vi "Host_Main.vi"() -> ()   [LabVIEW 2016]
uses:
  Application Control/FSM States.ctl
  Application Control/FSM Queue/FSM Data.ctl
  HostRTCommunication/Commands.ctl
  Raw Data/LoggingCommands.ctl
  Application Control/Application Globals.vi
panel:
  in  "Record Button":bool
  in  "Pause Button":bool
  in  "Configuration Cluster":T1={"Center Frequency"=50000000, "Sample Rate (Bandwidth)"=225001, "Tuner AGC Mode"=FALSE, "AGC Mode"=FALSE, "Manual Gain"=0, "Number of Averages"=4, "Frequency Correction"=0} {"Manual Gain" items=["0.000000", "0.900000", "1.400000", "2.700000", "3.700000", "7.700000", "8.700000", "12.500000", "14.400000", "15.700000", "16.600000", "19.700000", "20.700000", "22.900000", "25.400000", "28.000000", "29.700000", "32.800000", "33.800000", "36.400000", "37.200000", "38.600000", "40.200000", "42.100000", "43.400000", "43.900000", "44.500000", "48.000000", "49.600000"]; "Number of Averages" min=1 max=65536 step=1; "Sample Rate (Bandwidth)" min=225001 max=3200000 step=1; "Center Frequency" min=50000000 max=1800000000 step=1}
  in  "Connect":bool
  out "Spectrum Graph":dbl[](graph)
  out "Intensity Graph":dbl[][](graph)
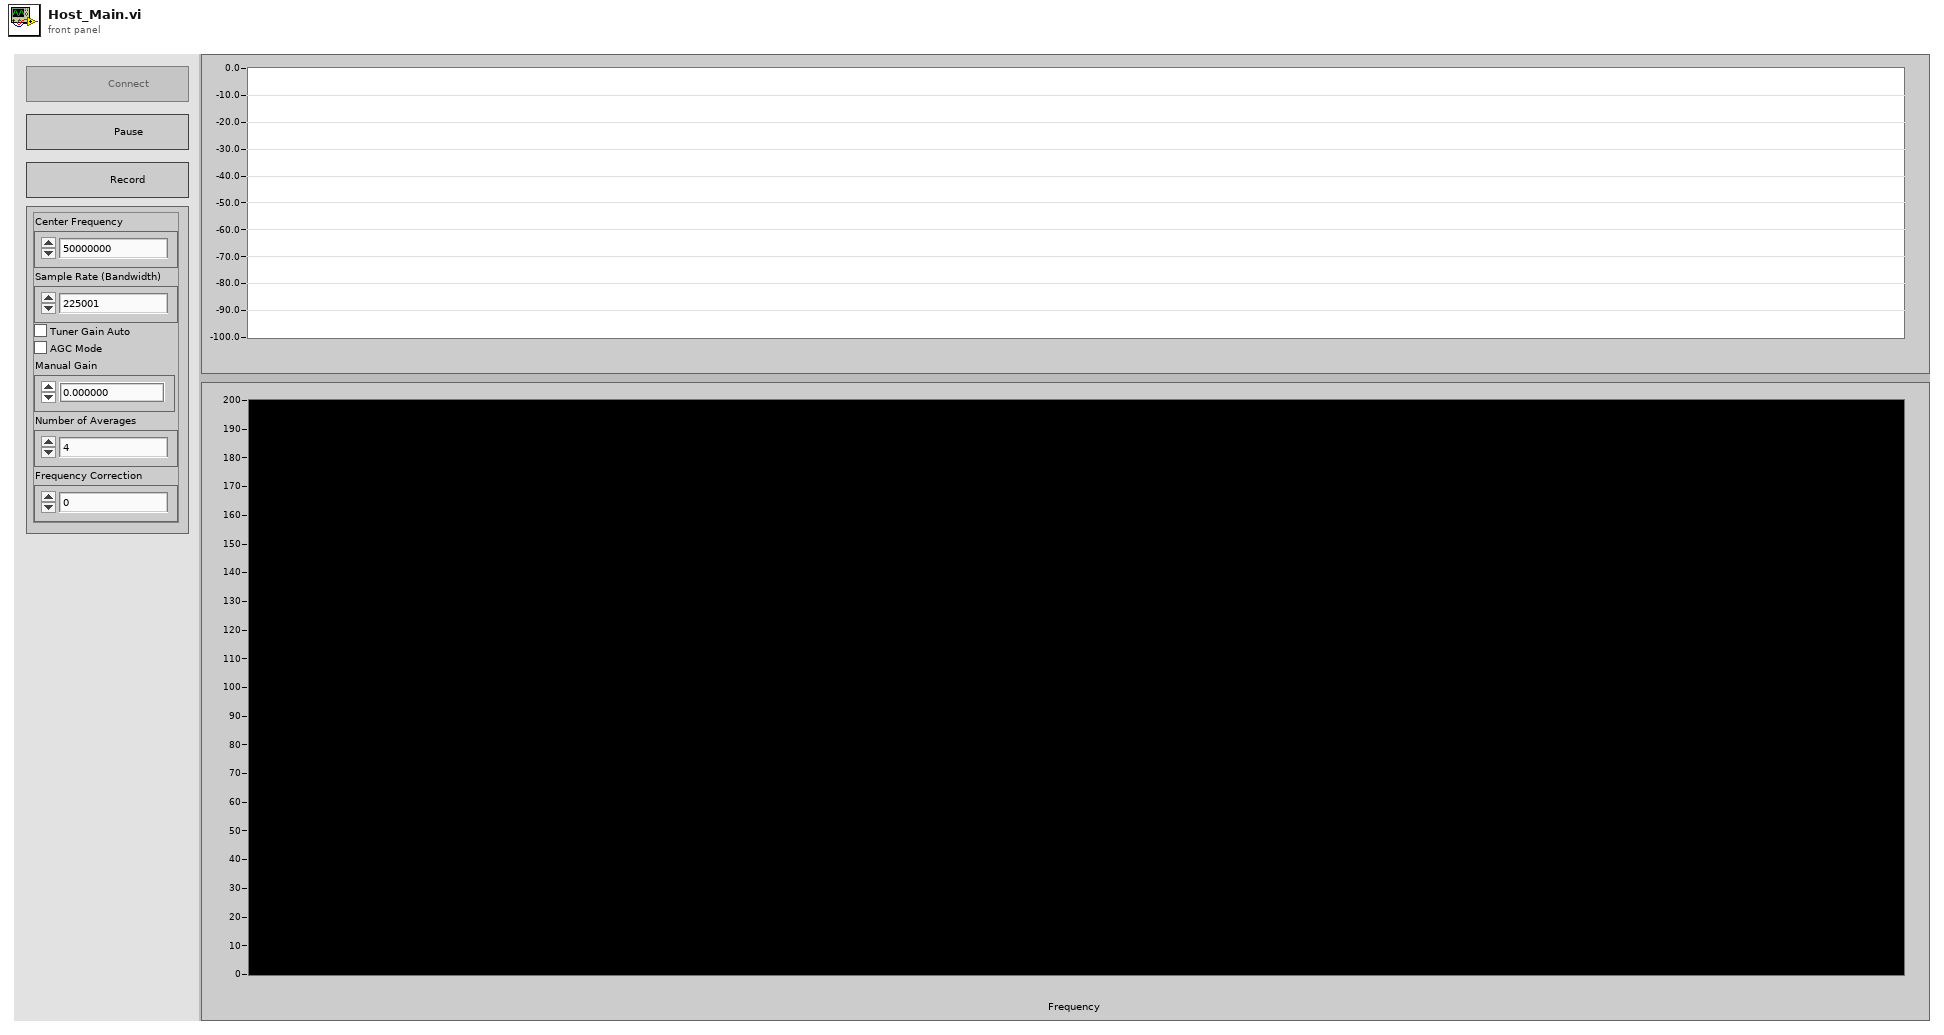
[diagram p1: front panel]
types:
  T1 = cluster{"Center Frequency":u32, "Sample Rate (Bandwidth)":u32, "Tuner AGC Mode":bool, "AGC Mode":bool, "Manual Gain":u16, "Number of Averages":u32, "Frequency Correction":i32}
  T2 = typedef "FSM Data.ctl" = cluster{"FSM State":T3, "Spectrum Reader":refnum<k21>, "Recording":bool, "IP Address":string, "Raw Data Reader":refnum<k21>}
  T3 = typedef "FSM States.ctl" = enum16{"App_Idle", "App_Connect", "App_Close", "APP_Init", "App_Logging", "App_SetRecordStateOn", "App_SetRecordStateOff"}
  T4 = enum8{"Enabled", "Disabled", "Disabled and Grayed Out"}
  T5 = typedef "LoggingCommands.ctl" = enum16{"Write", "Close File", "Open File", "Set Channel Metadata"}
  T6 = typedef "Commands.ctl" = enum16{"Set Center Frequency", "Set AGC State", "Set Number Of Averages", "Set Tuner Gain Mode", "Set Frequency Correction", "Set Sample Rate", "Set Manual Gain Value"}
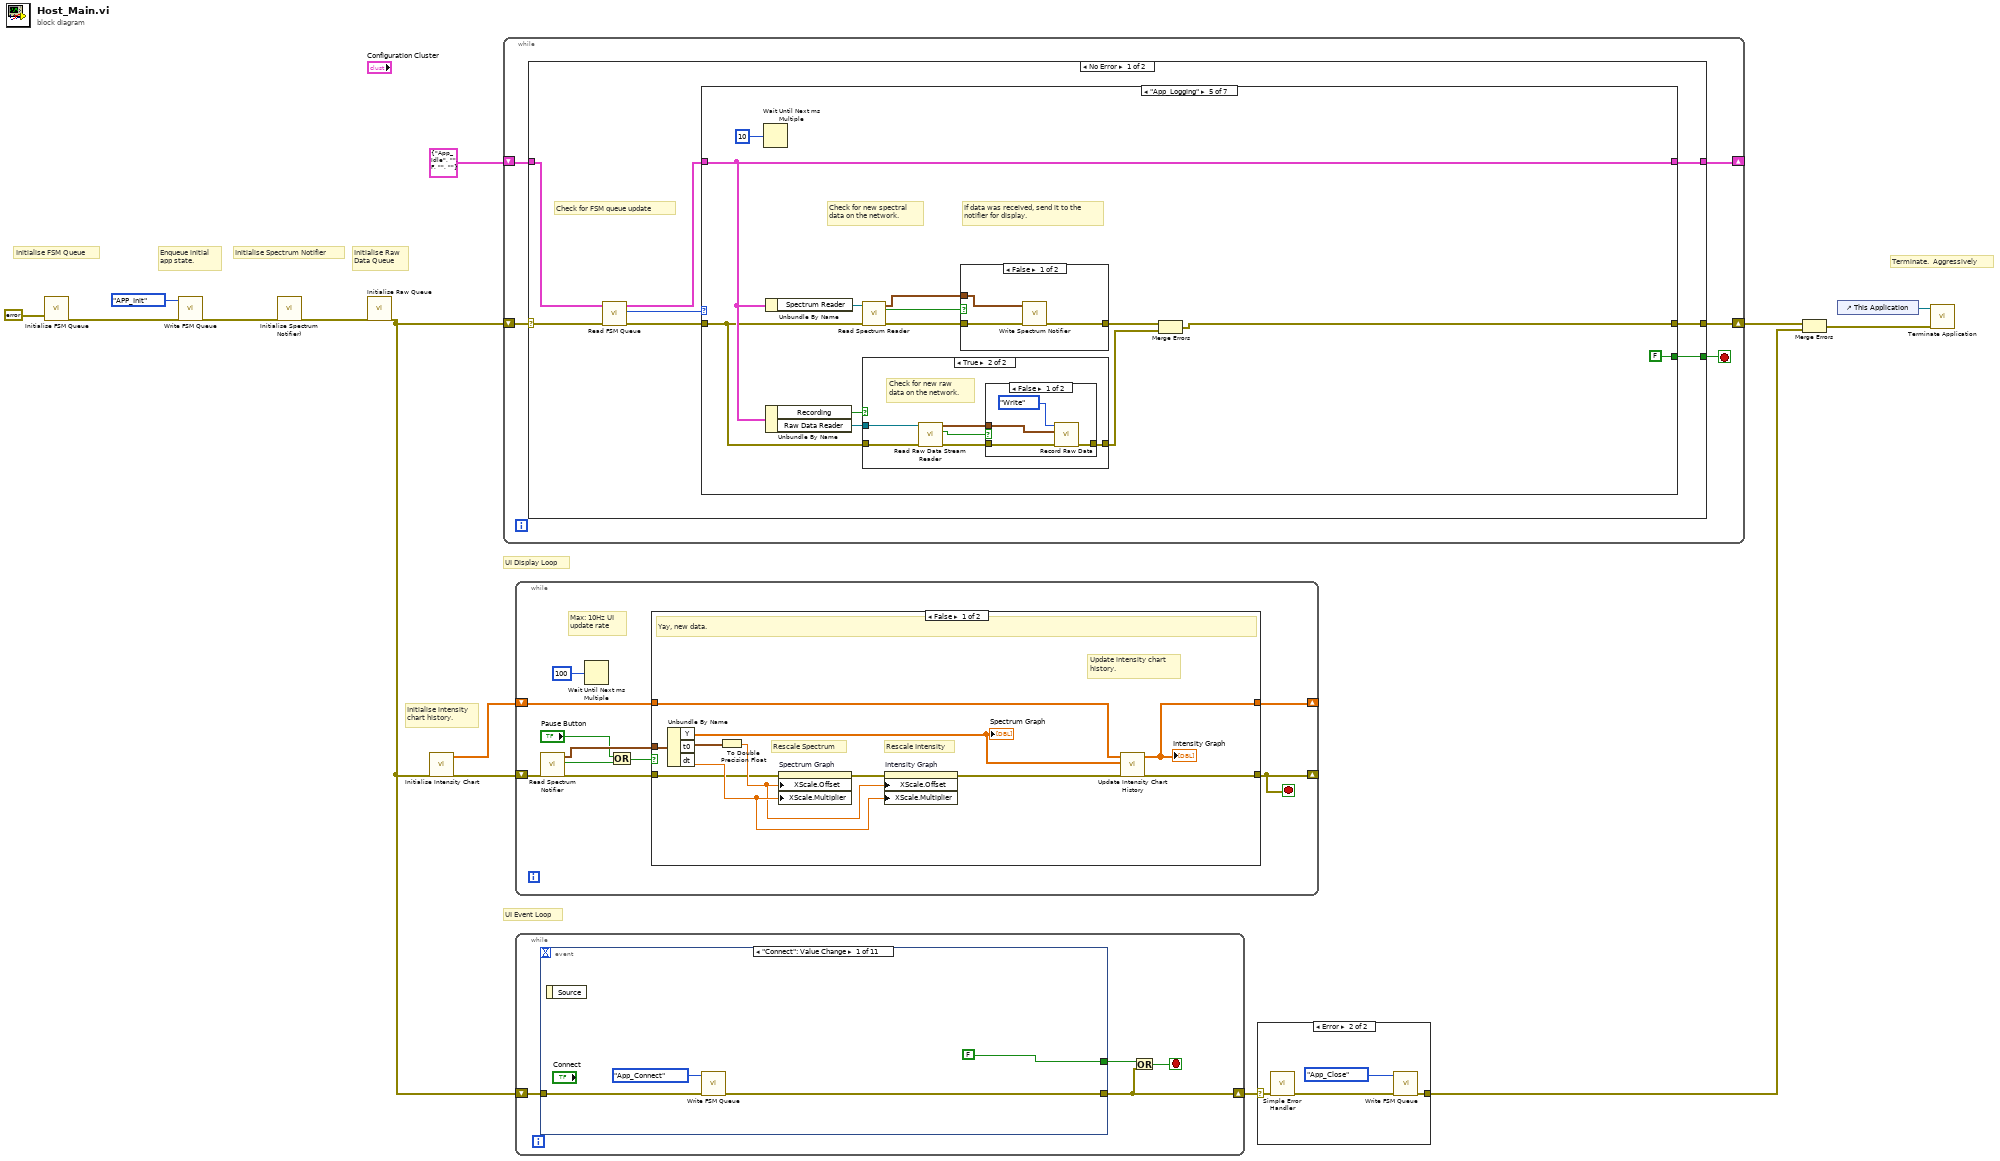
[diagram p0: block diagram]
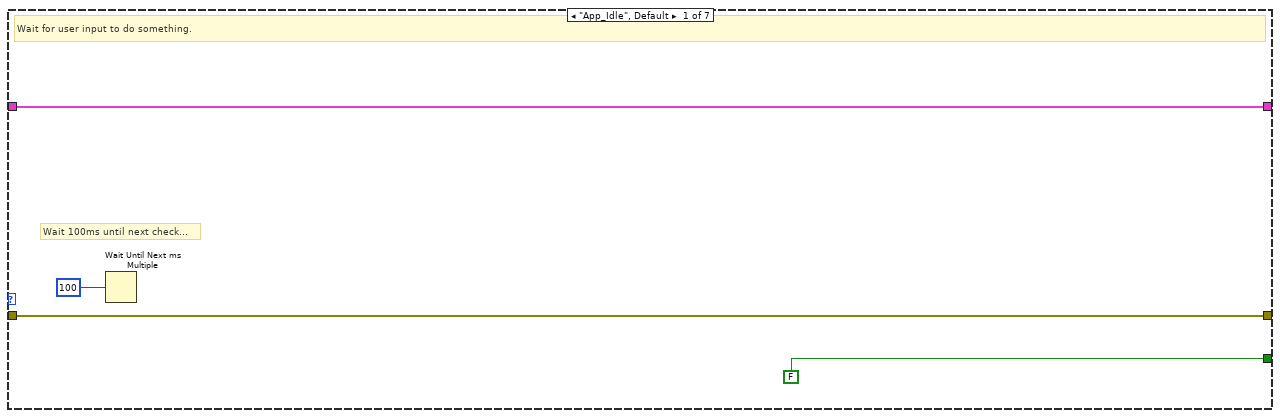
[diagram p2: hidden frame]
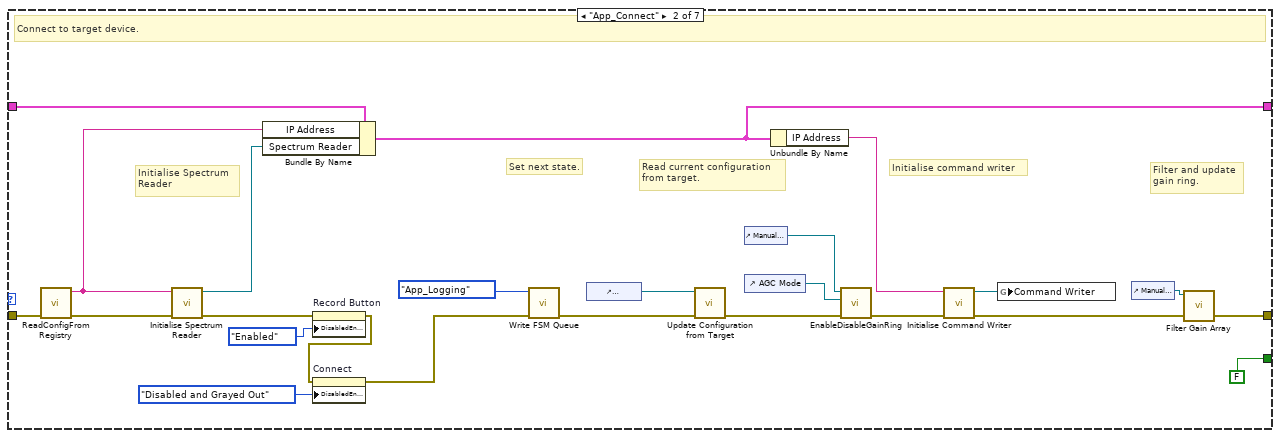
[diagram p3: hidden frame]
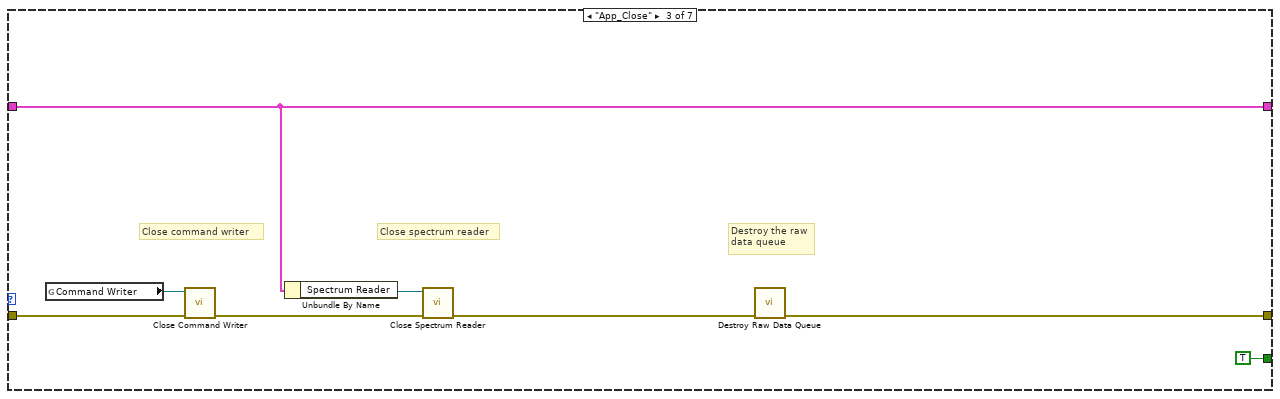
[diagram p4: hidden frame]
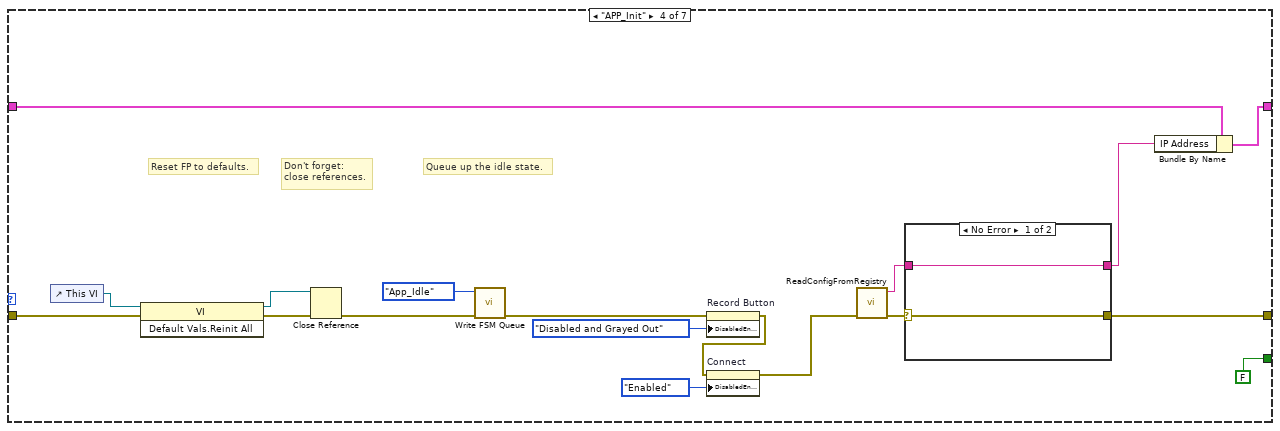
[diagram p5: hidden frame]
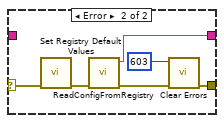
[diagram p6: hidden frame]
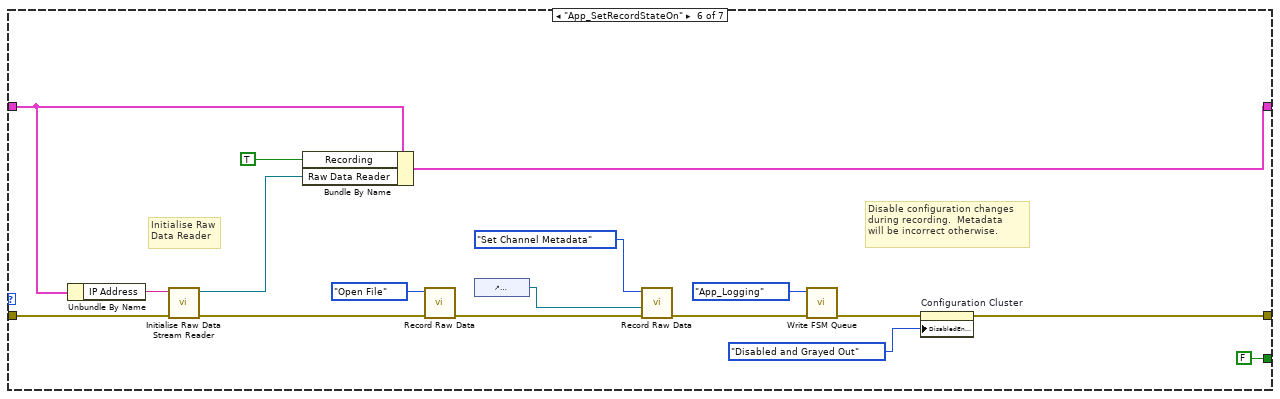
[diagram p10: hidden frame]
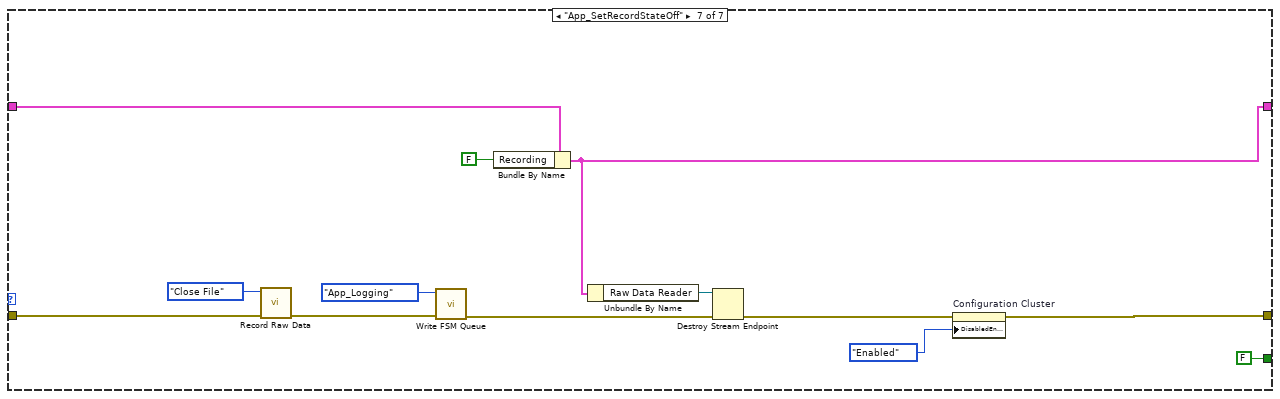
[diagram p11: hidden frame]
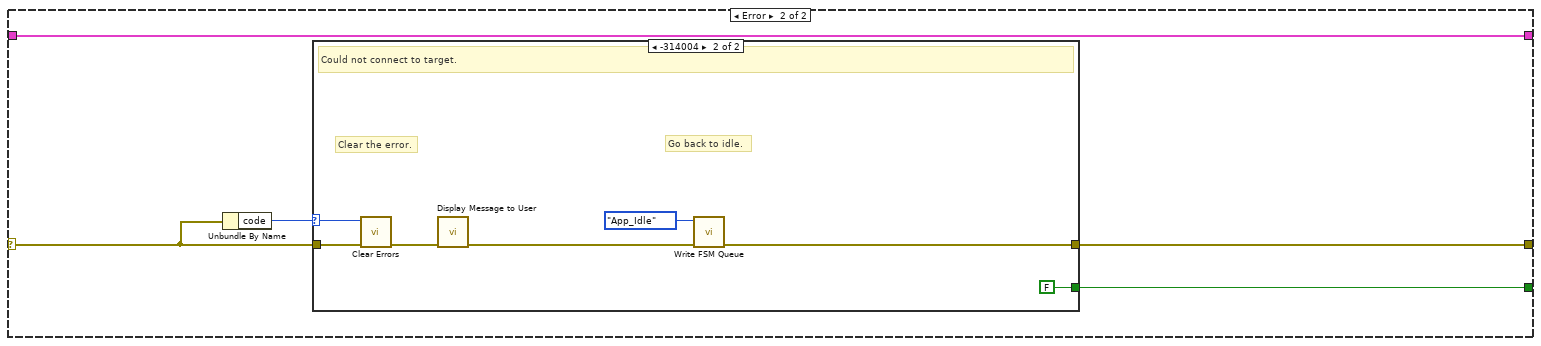
[diagram p12: hidden frame]
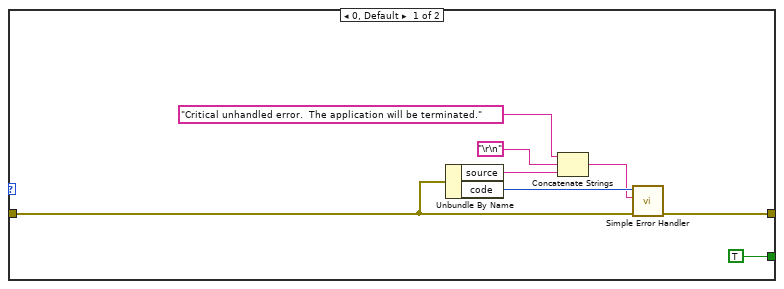
[diagram p13: hidden frame]
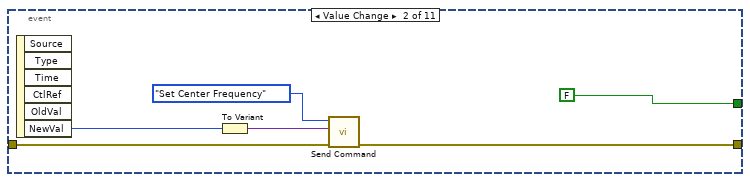
[diagram p16: hidden frame]
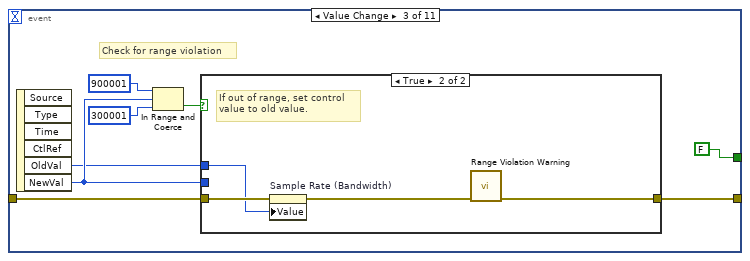
[diagram p17: hidden frame]
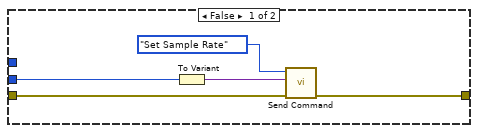
[diagram p18: hidden frame]
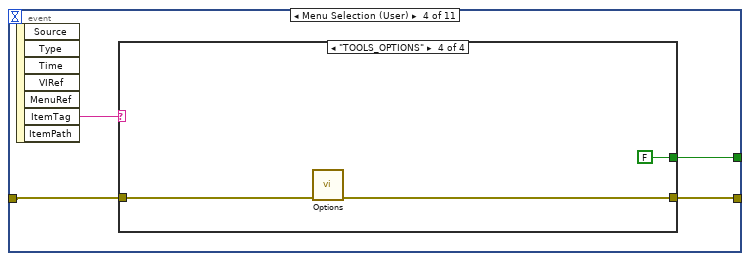
[diagram p19: hidden frame]
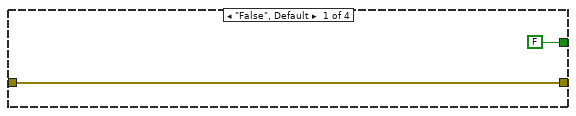
[diagram p20: hidden frame]
diagram:
  # "Initialise Raw\nData Queue"
  # "Initialise intensity\nchart history."
  # "UI Display Loop"
  # "Initialise Spectrum Notifier"
  # "Terminate.  Aggressively"
  # "Enqueue initial\napp state."
  # "Initialise FSM Queue"
  # "UI Event Loop"
  n1 = call "Initialise FSM Queue.vi"("error in (no error)"=errorcluster {"status"=FALSE, "code"=0, "source"=""}) -> ("error out"=w13:errorcluster)  [unwired: 10 in]
  n2 = call "Write FSM Queue.vi"("error in (no error)"=w13, "App_State"=FSM_States."APP_Init") -> ("error out"=w10:errorcluster)  [unwired: 9 in]
  n3 = call "Initialise Spectrum Notifier).vi"("error in (no error)"=w10) -> ("error out"=w3:errorcluster)  [unwired: 10 in]
  n4 = call "Initialise Raw Queue.vi"("error in (no error)"=w3) -> ("error out"=w1:errorcluster)  [unwired: 10 in]
  n5 = call "Initialise Intensity Chart.vi"("error in (no error)"=w1) -> ("error out"=w8:errorcluster, "Array"=w9:dbl[][])  [unwired: 9 in]
  n6 = while {
    shift-right: [w18] -> _
    shift-left: T2 {"FSM State"=enum."App_Idle", "Spectrum Reader"="", "Recording"=FALSE, "IP Address"="", "Raw Data Reader"=""} ("FSM Data") -> [w19]
    shift-right: [w17] -> w6
    shift-left: w1 -> [w16]
    stop <- w15 stop-if-true
    n7 = case shown="No Error" w16 {
      selector: w16 -> [w23 w151]
      tunnel: w19 -> [w27 w153]
      tunnel: [w21 w153] -> w18
      tunnel: [w24 w149] -> w17
      tunnel: [w20 w150] -> w15
      frame No Error {
        # "Check for FSM queue update"
        n8 = call "Read FSM Queue.vi"("error in (no error)"=w23, "FSM Data in"=w27) -> ("error out"=w25:errorcluster, "FSM State"=w26:T3, "FSM Data out"=w22:T2)  [unwired: 7 in]
        n9 = case shown="\"App_Logging\"" w26 {
          tunnel: w25 -> [w31 w36 w62 w79 w95 w131 w145]
          tunnel: [w31 w48 w57 w64 w92 w120 w136] -> w24
          tunnel: w22 -> [w30 w42 w58 w67 w97 w129 w147]
          tunnel: [w30 w33 w58 w65 w97 w134 w142] -> w21
          tunnel: [FALSE FALSE TRUE FALSE FALSE FALSE FALSE] -> w20
          frame "App_Idle", Default {
            # "Wait 100ms until next check..."
            # "Wait for user input to do something."
            n10 = Wait Until Next ms Multiple(millisecond multiple=u32 100) -> ()  [unwired: 1 out]
          }
          frame "App_Connect" {
            # "Initialise Spectrum \nReader"
            # "Filter and update\ngain ring."
            # "Initialise command writer"
            # "Read current configuration\nfrom target."
            # "Set next state."
            # "Connect to target device."
            n11 = call "ReadConfigFromRegistry.vi"("error in (no error)"=w36) -> ("error out"=w35:errorcluster, "String/Binary data"=w34:string)  [unwired: 9 in]
            n12 = call "Initialise Spectrum Reader.vi"("error in (no error)"=w35, "IP Address"=w34) -> ("error out"=w41:errorcluster, "Spectrum Reader"=w55:refnum<k21>)  [unwired: 8 in]
            n13 = Bundle By Name(cluster=w42, "IP Address"=w34, "Spectrum Reader"=w55) -> (w33:T2)
            n14 = property on="Record Button" class="Bool (strict)"(error in=w41, "DisabledEnum"=T4."Enabled" ("Disabled")) -> (error out=w38:errorcluster)  [unwired: 1 in, 1 out]
            n15 = property on="Connect" class="Bool"(error in=w38, "DisabledEnum"=T4."Disabled and Grayed Out" ("Disabled")) -> (error out=w37:errorcluster)  [unwired: 1 in, 1 out]
            n16 = call "Write FSM Queue.vi"("error in (no error)"=w37, "App_State"=FSM_States."App_Logging") -> ("error out"=w52:errorcluster)  [unwired: 9 in]
            n17 = control-ref of="Configuration Cluster"() -> (w50:refnum<vi>)
            n18 = call "Update Configuration from Target.vi"("error in (no error)"=w52, "Configuration Cluster"=w50) -> ("error out"=w46:errorcluster)  [unwired: 9 in]
            n19 = control-ref of="Manual Gain"() -> (w44:refnum<vi>)
            n20 = control-ref of="AGC Mode"() -> (w43:refnum<vi>)
            n21 = Unbundle By Name(w33) -> ("IP Address"=w32:string)
            n22 = call "EnableDisableGainRing.vi"("error in (no error)"=w46, "Bool Refnum"=w43, "Ring in"=w44) -> ("error out"=w45:errorcluster)  [unwired: 8 in]
            n23 = call "Initialise Command Writer.vi"("error in (no error)"=w45, "IP Address"=w32) -> ("error out"=w49:errorcluster, "Refnum out"=w51:refnum<k21>)  [unwired: 8 in]
            n24 = global write "Application Globals.vi" "Command Writer"(w51) -> ()
            n25 = control-ref of="Manual Gain"() -> (w47:refnum<vi>)
            n26 = call "Filter Gain Array.vi"("error in (no error)"=w49, "Gain Ring Reference"=w47) -> ("error out"=w48:errorcluster)  [unwired: 9 in]
          }
          frame "App_Close" {
            # "Destroy the raw\ndata queue"
            # "Close spectrum reader"
            # "Close command writer"
            n27 = global read "Application Globals.vi" "Command Writer"() -> (w61:refnum<k21>)
            n28 = call "Close Command Writer.vi"("error in (no error)"=w62, "Refnum in"=w61) -> ("error out"=w60:errorcluster)  [unwired: 9 in]
            n29 = Unbundle By Name(w58) -> ("Spectrum Reader"=w59:refnum<k21>)
            n30 = call "Close Spectrum Reader.vi"("error in (no error)"=w60, "endpoint in"=w59) -> ("error out"=w56:errorcluster)  [unwired: 9 in]
            n31 = call "Destroy Raw Data Queue.vi"("error in (no error)"=w56) -> ("error out"=w57:errorcluster)  [unwired: 10 in]
          }
          frame "APP_Init" {
            # "Queue up the idle state."
            # "Don't forget:\nclose references."
            # "Reset FP to defaults."
            n32 = control-ref of="This VI"() -> (w80:refnum<vi>)
            n33 = invoke class="VI" method="Default Vals.Reinit All"(reference=w80, error in=w79) -> (reference out=w76:refnum<vi>, error out=w78:errorcluster)  [unwired: 1 in, 1 out]
            n34 = Close Reference(reference=w76, error in (no error)=w78) -> (error out=w77:errorcluster)
            n35 = call "Write FSM Queue.vi"("error in (no error)"=w77, "App_State"=FSM_States."App_Idle") -> ("error out"=w74:errorcluster)  [unwired: 9 in]
            n36 = property on="Record Button" class="Bool (strict)"(error in=w74, "DisabledEnum"=T4."Disabled and Grayed Out" ("Disabled")) -> (error out=w72:errorcluster)  [unwired: 1 in, 1 out]
            n37 = property on="Connect" class="Bool"(error in=w72, "DisabledEnum"=T4."Enabled" ("Disabled")) -> (error out=w69:errorcluster)  [unwired: 1 in, 1 out]
            n38 = call "ReadConfigFromRegistry.vi"("error in (no error)"=w69) -> ("error out"=w70:errorcluster, "String/Binary data"=w68:string)  [unwired: 9 in]
            n39 = case shown="No Error" w70 {
              selector: w70 -> [w82 w89]
              tunnel: [w83 w87] -> w66
              tunnel: w68 -> [w83 _]
              tunnel: [w82 w84] -> w64
              frame No Error {
              }
              frame Error {
                n40 = call "Set Registry Default Values.vi"("error in (no error)"=w89) -> ("error out"=w88:errorcluster)  [unwired: 10 in]
                n41 = call "ReadConfigFromRegistry.vi"("error in (no error)"=w88) -> ("error out"=w86:errorcluster, "String/Binary data"=w87:string)  [unwired: 9 in]
                n42 = call <vilib>:"Clear Errors.vi"("error in (no error)"=w86, "specific error code to clear (0: all)"=603) -> ("error out"=w84:errorcluster)  [unwired: 4 in, 1 out]
              }
            }
            n43 = Bundle By Name(cluster=w67, "IP Address"=w66) -> (w65:T2)
          }
          frame "App_Logging" {
            # "If data was received, send it to the\nnotifier for display."
            # "Check for new spectral\ndata on the network."
            n44 = Wait Until Next ms Multiple(millisecond multiple=u32 10) -> ()  [unwired: 1 out]
            n45 = Unbundle By Name(w97) -> ("Spectrum Reader"=w102:refnum<k21>)
            n46 = Unbundle By Name(w97) -> ("Recording"=w90:bool, "Raw Data Reader"=w96:refnum<k21>)
            n47 = call "Read Spectrum Reader.vi"("error in (no error)"=w95, "Refnum in"=w102) -> ("error out"=w99:errorcluster, "Boolean"=w100:bool, "output waveform"=w98:waveform(dbl))  [unwired: 7 in]
            n48 = case shown="True" w90 {
              tunnel: w96 -> [_ w109]
              tunnel: w95 -> [w103 w108]
              tunnel: [w103 w106] -> w93
              frame False {
              }
              frame True {
                # "Check for new raw\ndata on the network."
                n49 = call "Read Raw Data Stream Reader.vi"("error in (no error)"=w108, "Raw Data Reader"=w109) -> ("error out"=w107:errorcluster, "timed out?"=w104:bool, "Output Waveform"=w105:waveform(u8))  [unwired: 7 in]
                n50 = case shown="False" w104 {
                  tunnel: w107 -> [w113 w114]
                  tunnel: [w112 w114] -> w106
                  tunnel: w105 -> [w111 _]
                  frame False {
                    n51 = call "Record Raw Data.vi"("error in (no error)"=w113, "Raw Data"=w111, "Command"=LoggingCommands."Write") -> ("error out"=w112:errorcluster)  [unwired: 8 in]
                  }
                  frame True {
                  }
                }
              }
            }
            n52 = case shown="False" w100 {
              tunnel: [w117 w118] -> w94
              tunnel: w99 -> [w115 w118]
              tunnel: w98 -> [w116 _]
              frame False {
                n53 = call "Write Spectrum Notifier.vi"("error in (no error)"=w115, "Waveform"=w116) -> ("error out"=w117:errorcluster)  [unwired: 9 in]
              }
              frame True {
              }
            }
            n54 = Merge Errors(w94, w93) -> (w92:errorcluster)
          }
          frame "App_SetRecordStateOn" {
            # "Disable configuration changes\nduring recording.  Metadata\nwill be incorrect otherwise."
            # "Initialise Raw\nData Reader"
            n55 = Unbundle By Name(w129) -> ("IP Address"=w128:string)
            n56 = call "Initialise Raw Data Stream Reader.vi"("error in (no error)"=w131, "IP Address"=w128) -> ("error out"=w130:errorcluster, "reader endpoint"=w127:refnum<k21>)  [unwired: 8 in]
            n57 = Bundle By Name(cluster=w129, "Recording"=TRUE, "Raw Data Reader"=w127) -> (w134:T2)
            n58 = call "Record Raw Data.vi"("error in (no error)"=w130, "Command"=LoggingCommands."Open File") -> ("error out"=w125:errorcluster)  [unwired: 9 in]
            n59 = control-ref of="Configuration Cluster"() -> (w122:refnum<vi>)
            n60 = call "Record Raw Data.vi"("error in (no error)"=w125, "Configuration Cluster"=w122, "Command"=LoggingCommands."Set Channel Metadata") -> ("error out"=w124:errorcluster)  [unwired: 8 in]
            n61 = call "Write FSM Queue.vi"("error in (no error)"=w124, "App_State"=FSM_States."App_Logging") -> ("error out"=w121:errorcluster)  [unwired: 9 in]
            n62 = property on="Configuration Cluster" class="Clust (strict)"(error in=w121, "DisabledEnum"=T4."Disabled and Grayed Out" ("Disabled")) -> (error out=w120:errorcluster)  [unwired: 1 in, 1 out]
          }
          frame "App_SetRecordStateOff" {
            n63 = call "Record Raw Data.vi"("error in (no error)"=w145, "Command"=LoggingCommands."Close File") -> ("error out"=w144:errorcluster)  [unwired: 9 in]
            n64 = call "Write FSM Queue.vi"("error in (no error)"=w144, "App_State"=FSM_States."App_Logging") -> ("error out"=w141:errorcluster)  [unwired: 9 in]
            n65 = Bundle By Name(cluster=w147, "Recording"=FALSE) -> (w142:T2)
            n66 = Unbundle By Name(w142) -> ("Raw Data Reader"=w140:refnum<k21>)
            n67 = Destroy Stream Endpoint(8:w141, 11:w140) -> (0:w137:errorcluster)
            n68 = property on="Configuration Cluster" class="Clust (strict)"(error in=w137, "DisabledEnum"=T4."Enabled" ("Disabled")) -> (error out=w136:errorcluster)  [unwired: 1 in, 1 out]
          }
        }
      }
      frame Error {
        n69 = Unbundle By Name(w151) -> ("code"=w152:i32)
        n70 = case shown="-314004" w152 {
          selector: w152 -> [_ w166]
          tunnel: w151 -> [w160 w167]
          tunnel: [TRUE FALSE] -> w150
          tunnel: [w154 w162] -> w149
          frame 0, Default {
            n71 = Unbundle By Name(w160) -> ("source"=w158:string, "code"=w159:i32)
            n72 = Concatenate Strings("Critical unhandled error.  The application will be terminated.", "\r\n", w158) -> (w155:string)
            n73 = call <vilib>:"Simple Error Handler.vi"("error code (no error:0)"=w159, "error source (\" \")"=w155, "error in (no error)"=w160) -> ("error out"=w154:errorcluster)  [unwired: 2 in, 4 out]
          }
          frame -314004 {
            # "Go back to idle."
            # "Clear the error."
            # "Could not connect to target."
            n74 = call <vilib>:"Clear Errors.vi"("error in (no error)"=w167, "specific error code to clear (0: all)"=w166) -> ("error out"=w165:errorcluster)  [unwired: 4 in, 1 out]
            n75 = call "Display Message to User"("error in (no error)"=w165) -> ("error out"=w163:errorcluster)  [unwired: 9 in, 1 out]
            n76 = call "Write FSM Queue.vi"("error in (no error)"=w163, "App_State"=FSM_States."App_Idle") -> ("error out"=w162:errorcluster)  [unwired: 9 in]
          }
        }
      }
    }
  }
  n77 = while {
    shift-right: [w172] -> _
    shift-left: w8 -> [w178]
    shift-right: [w174] -> _
    shift-left: w9 -> [w175]
    stop <- w172 stop-if-true
    # "Max: 10Hz UI \nupdate rate"
    n78 = call "Read Spectrum Notifier.vi"("error in (no error)"=w178) -> ("error out"=w177:errorcluster, "timed out?"=w171:bool, "WaveForm Out"=w176:waveform(dbl))  [unwired: 8 in]
    n79 = Wait Until Next ms Multiple(millisecond multiple=u32 100) -> ()  [unwired: 1 out]
    n80 = Or(x="Pause Button", y=w171) -> (x .or. y?=w170:bool)
    n81 = case shown="False" w170 {
      tunnel: [w186 w191] -> w172
      tunnel: w177 -> [w180 w191]
      tunnel: w176 -> [w189 _]
      tunnel: w175 -> [w188 w190]
      tunnel: [w187 w190] -> w174
      frame False {
        # "Rescale Intensity"
        # "Rescale Spectrum"
        # "Update intensity chart\nhistory."
        # "Yay, new data."
        n82 = Unbundle By Name(w189) -> ("Y"=w179:dbl[], "t0"=w184:timestamp, "dt"=w183:dbl)
        "Spectrum Graph" <- w179
        n83 = To Double Precision Float(number=w184) -> (double precision float=w182:dbl)
        n84 = property on="Spectrum Graph" class="WFGraph (strict)"(error in=w180, "XScale.Offset"=w182, "XScale.Multiplier"=w183) -> (error out=w181:errorcluster)  [unwired: 1 in, 1 out]
        n85 = property on="Intensity Graph" class="IntGraph (strict)"(error in=w181, "XScale.Offset"=w182, "XScale.Multiplier"=w183) -> (error out=w185:errorcluster)  [unwired: 1 in, 1 out]
        n86 = call "Update Intensity Chart History.vi"("error in (no error)"=w185, "Y"=w179, "Array in"=w188) -> ("error out"=w186:errorcluster, "Array out"=w187:dbl[][])  [unwired: 7 in]
        "Intensity Graph" <- w187
      }
      frame True {
        # "Timeout is true.  No new data received."
      }
    }
  }
  n87 = while {
    shift-right: [w192] -> w7
    shift-left: w1 -> [w195]
    stop <- w193 stop-if-true
    n88 = event shown="[0] \"Connect\": Value Change" {
      selector: _ -> [_ _ _ _ _ _ _ _ _ _ _]
      dyn-events: _ -> [_ _ _ _ _ _ _ _ _ _ _]
      timeout: _ -> [_ _ _ _ _ _ _ _ _ _ _]
      tunnel: [FALSE ("Discard?") FALSE ("Discard?") FALSE ("Discard?") w225 FALSE ("Discard?") FALSE ("Discard?") FALSE ("Discard?") FALSE ("Discard?") FALSE ("Discard?") w282 FALSE ("Discard?")] -> w194
      tunnel: w195 -> [w197 w202 w213 w224 w244 w251 w266 w270 w275 w280 w286]
      tunnel: [w196 w201 w212 w223 w239 w250 w257 w269 w276 w279 w285] -> w192
      event "Connect": Value Change {
        n89 = event-data() -> ()  [unwired: 1 in, 1 out]
        n90 = call "Write FSM Queue.vi"("error in (no error)"=w197, "App_State"=FSM_States."App_Connect") -> ("error out"=w196:errorcluster)  [unwired: 9 in]
      }
      event "Configuration Cluster.Center Frequency": Value Change {
        n91 = event-data() -> ("NewVal"=w200:u32)  [unwired: 1 in, 5 out]
        n92 = To Variant(anything=w200) -> (Variant=w204:variant)
        n93 = call "Send Command.vi"("error in (no error)"=w202, "Parameter"=w204, "Command"=Commands."Set Center Frequency") -> ("error out"=w201:errorcluster)  [unwired: 8 in]
      }
      event "Configuration Cluster.Sample Rate (Bandwidth)": Value Change {
        # "Check for range violation"
        n94 = event-data() -> ("OldVal"=w206:u32, "NewVal"=w210:u32)  [unwired: 1 in, 4 out]
        n95 = In Range and Coerce(upper limit=u32 900001, x=w210, lower limit=u32 300001) -> (In Range?=w207:bool)  [unwired: 1 out]
        n96 = case shown="True" w207 {
          tunnel: w213 -> [w216 w222]
          tunnel: [w215 w219] -> w212
          tunnel: w210 -> [w214 _]
          tunnel: w206 -> [_ w221]
          frame False {
            n97 = To Variant(anything=w214) -> (Variant=w217:variant)
            n98 = call "Send Command.vi"("error in (no error)"=w216, "Parameter"=w217, "Command"=Commands."Set Sample Rate") -> ("error out"=w215:errorcluster)  [unwired: 8 in]
          }
          frame True {
            # "If out of range, set control \nvalue to old value."
            n99 = property on="Sample Rate (Bandwidth)" class="DigNum (strict)"(error in=w222, "Value"=w221) -> (error out=w220:errorcluster)  [unwired: 1 in, 1 out]
            n100 = call "Range Violation Warning"("error in (no error)"=w220) -> ("error out"=w219:errorcluster)  [unwired: 9 in, 1 out]
          }
        }
      }
      event Menu Selection (User) {
        n101 = event-data() -> ("ItemTag"=w226:string)  [unwired: 1 in, 6 out]
        n102 = case shown="\"TOOLS_OPTIONS\"" w226 {
          tunnel: [FALSE TRUE FALSE FALSE] -> w225
          tunnel: w224 -> [w227 w230 w235 w238]
          tunnel: [w227 w229 w234 w237] -> w223
          frame "False", Default {
          }
          frame "APP_EXIT" {
            # "Signal application exit..."
            n103 = call "Write FSM Queue.vi"("error in (no error)"=w230, "App_State"=FSM_States."App_Close") -> ("error out"=w229:errorcluster)  [unwired: 9 in]
          }
          frame "HELP_ABOUT" {
            # "Show \"about\" dialog\""
            n104 = call "About.vi"("error in (no error)"=w235) -> ("error out"=w234:errorcluster)  [unwired: 10 in]
          }
          frame "TOOLS_OPTIONS" {
            n105 = call "Options.vi"("error in (no error)"=w238) -> ("error out"=w237:errorcluster)  [unwired: 10 in]
          }
        }
      }
      event "Configuration Cluster.Tuner AGC Mode": Value Change {
        n106 = event-data() -> ("NewVal"=w242:bool)  [unwired: 1 in, 5 out]
        n107 = case shown="False" w242 {
          tunnel: [T4."Enabled" ("Disabled") T4."Disabled and Grayed Out" ("Disabled")] -> w241
          frame False {
          }
          frame True {
          }
        }
        n108 = To Variant(anything=w242) -> (Variant=w245:variant)
        n109 = call "Send Command.vi"("error in (no error)"=w244, "Parameter"=w245, "Command"=Commands."Set Tuner Gain Mode") -> ("error out"=w240:errorcluster)  [unwired: 8 in]
        n110 = property on="Manual Gain" class="Ring (strict)"(error in=w240, "DisabledEnum"=w241) -> (error out=w239:errorcluster)  [unwired: 1 in, 1 out]
      }
      event "Record Button": Value Change {
        n111 = event-data() -> ("NewVal"=w253:bool)  [unwired: 1 in, 5 out]
        n112 = case shown="True" w253 {
          tunnel: [FSM_States."App_SetRecordStateOff" ("App_State") FSM_States."App_SetRecordStateOn" ("App_State")] -> w252
          frame False {
          }
          frame True {
          }
        }
        n113 = call "Write FSM Queue.vi"("error in (no error)"=w251, "App_State"=w252) -> ("error out"=w250:errorcluster)  [unwired: 9 in]
      }
      event "Configuration Cluster.Manual Gain": Value Change {
        n114 = event-data() -> ("NewVal"=w264:u16)  [unwired: 1 in, 5 out]
        n115 = property on="Manual Gain" class="Ring (strict)"(error in=w266) -> (error out=w261:errorcluster, "Strings []"=w265:string[])  [unwired: 1 in, 1 out]
        n116 = Index Array(array=w265, index=w264) -> (element=w258:string)
        n117 = Fract/Exp String To Number(use system decimal point (T)=FALSE, string=w258) -> (number=w260:dbl)  [unwired: 2 in, 1 out]
        n118 = To Variant(anything=w260) -> (Variant=w262:variant)
        n119 = call "Send Command.vi"("error in (no error)"=w261, "Parameter"=w262, "Command"=Commands."Set Manual Gain Value") -> ("error out"=w257:errorcluster)  [unwired: 8 in]
      }
      event "Configuration Cluster.AGC Mode": Value Change {
        n120 = event-data() -> ("NewVal"=w267:bool)  [unwired: 1 in, 5 out]
        n121 = To Variant(anything=w267) -> (Variant=w271:variant)
        n122 = call "Send Command.vi"("error in (no error)"=w270, "Parameter"=w271, "Command"=Commands."Set AGC State") -> ("error out"=w269:errorcluster)  [unwired: 8 in]
      }
      event "Configuration Cluster.Frequency Correction": Value Change {
        n123 = event-data() -> ("NewVal"=w274:i32)  [unwired: 1 in, 5 out]
        n124 = To Variant(anything=w274) -> (Variant=w277:variant)
        n125 = call "Send Command.vi"("error in (no error)"=w275, "Parameter"=w277, "Command"=Commands."Set Frequency Correction") -> ("error out"=w276:errorcluster)  [unwired: 8 in]
      }
      event Panel Close? {
        w282 = TRUE ("Discard?")
        n126 = event-data() -> ()  [unwired: 1 in, 4 out]
        n127 = call "Write FSM Queue.vi"("error in (no error)"=w280, "App_State"=FSM_States."App_Close") -> ("error out"=w279:errorcluster)  [unwired: 9 in]
        n128 = event-data("Discard?"=w282) -> ()  [unwired: 1 in, 1 out]
      }
      event "Configuration Cluster.Number of Averages": Value Change {
        n129 = event-data() -> ("NewVal"=w283:u32)  [unwired: 1 in, 5 out]
        n130 = To Variant(anything=w283) -> (Variant=w287:variant)
        n131 = call "Send Command.vi"("error in (no error)"=w286, "Parameter"=w287, "Command"=Commands."Set Number Of Averages") -> ("error out"=w285:errorcluster)  [unwired: 8 in]
      }
    }
    n132 = Or(x=w194, y=w192) -> (x .or. y?=w193:bool)
  }
  n133 = case shown="Error" w7 {
    selector: w7 -> [w289 w293]
    tunnel: [w289 w290] -> w5
    frame No Error {
    }
    frame Error {
      n134 = call <vilib>:"Simple Error Handler.vi"("error in (no error)"=w293) -> ("error out"=w291:errorcluster)  [unwired: 4 in, 4 out]
      n135 = call "Write FSM Queue.vi"("error in (no error)"=w291, "App_State"=FSM_States."App_Close") -> ("error out"=w290:errorcluster)  [unwired: 9 in]
    }
  }
  n136 = Merge Errors(w6, w5) -> (w4:errorcluster)
  n137 = control-ref of="This Application"() -> (w11:refnum<vi>)
  n138 = call "Terminate Application.vi"("error in (no error)"=w4, "Application in"=w11) -> ()  [unwired: 10 in]
